vi "gate valve test (inproj).vi"() -> ()   [LabVIEW 2013]
uses:
  <vilib>/DAQmx/write.llb/DAQmx Write.vi
  <vilib>/DAQmx/write.llb/DAQmx Write (Digital Bool 1Line 1Point).vi
  <vilib>/DAQmx/miscellaneous.llb/DAQmx Fill In Error Info.vi
panel:
  in  "Boolean":bool
  out "GV Status":bool
  in  "stop":bool
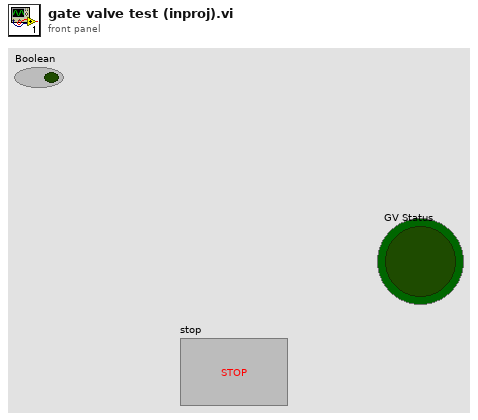
[diagram p1: front panel]
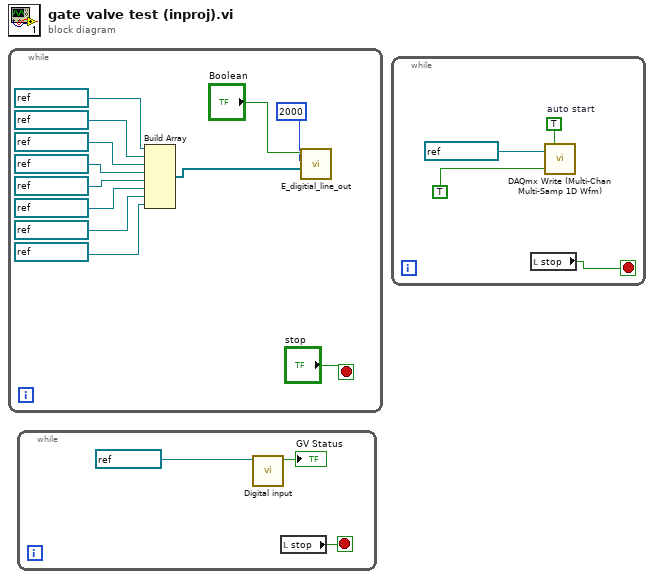
[diagram p0: block diagram]
diagram:
  n1 = while {
    stop <- "stop" stop-if-true
    n2 = Build Array(refnum<k21> "P0L0 out" ("task/channels in"), refnum<k21> "P0L1 out" ("task/channels in"), refnum<k21> "P0L2 out" ("task/channels in"), refnum<k21> "P0L3 out" ("task/channels in"), refnum<k21> "P0L4 out" ("task/channels in"), refnum<k21> "P0L5 out" ("task/channels in"), refnum<k21> "P0L6 out" ("task/channels in"), refnum<k21> "P0L7 out" ("element")) -> (w3:refnum<k21>[])
    n3 = call "E_digitial_line_out.vi"("Array"=w3, "milliseconds to wait"=u32 2000, "Boolean"="Boolean") -> ()  [unwired: 3 in, 1 out]
  }
  n4 = while {
    stop <- w15 stop-if-true
    n5 = call "Digital input.vi"("task/channels in"=refnum<k21> "P0L8 in") -> ("element 2"=→"GV Status":bool)  [unwired: 9 in, 1 out]
    n6 = local read "stop"() -> (w15:bool)
  }
  n7 = while {
    stop <- w19 stop-if-true
    w17 = TRUE  # auto start
    n8 = local read "stop"() -> (w19:bool)
    n9 = call-poly "DAQmx Write (Multi-Chan Multi-Samp 1D Wfm).vi"("task/channels in"=refnum<k21> "P0L2 out", "auto start"=w17, "data"=TRUE ("Button 1 \n(relay 1 engage) 2")) -> ()  [unwired: 10 in, 3 out]
  }
